vi "Search_comm_map_and_interrogate.vi"(7 "array of registers":T2[](array[typedef]) {"Cluster"."Mode" items=["None", "MODBUS", "HART", "Profibus DP", "Profibus PA", "Fieldbus", "DeviceNET"]}, 8 "error in (no error)":errorcluster, 9 "Register name":string="Flow Calibration Factor", 11 "Protocol in":refnum<class "Protocol.lvclass">) -> (0 "error out":errorcluster, 3 "Protocol out":refnum<class "Protocol.lvclass">, 4 "output cluster":T1)   [LabVIEW 2016]
uses:
  Typedef/comm_variable_definition.ctl
  Typedef/Comm_mode_and_address_type.ctl
  Typedef/Comm_mode_type_combo.ctl
  Protocol Class/Protocol.lvclass
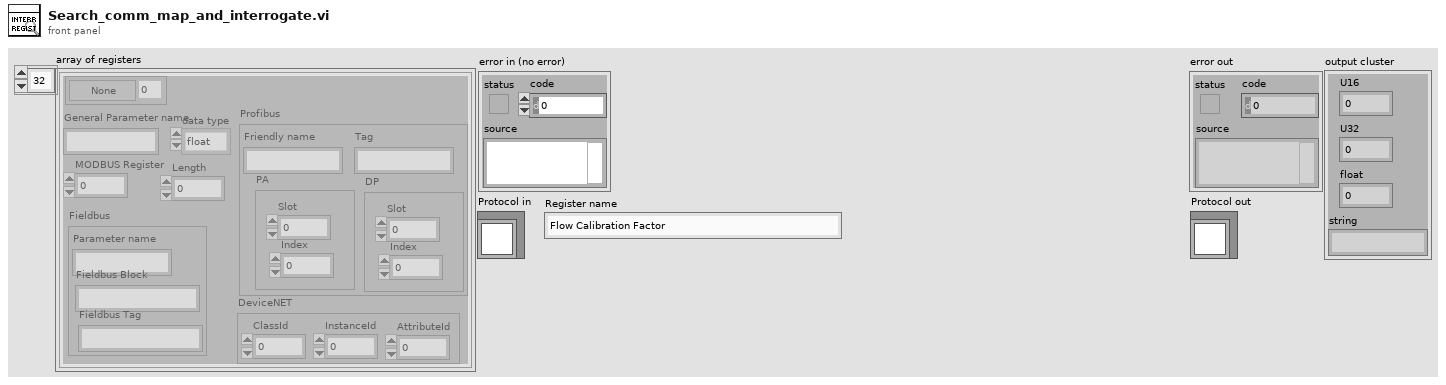
[diagram p1: front panel]
types:
  T1 = cluster{"U16":u16, "U32":u32, "float":sgl, "string":string}
  T2 = typedef "comm_variable_definition.ctl" = cluster{"General Parameter name":string, "MODBUS Register":i32, "Profibus":cluster{"Friendly name":string, "PA":cluster{"Slot":i32, "Index":i32}, "DP":cluster{"Slot":i32, "Index":i32}, "Tag":string}, "Fieldbus":cluster{"Parameter name":string, "Fieldbus Block":string, "Fieldbus Tag":string}, "data type":enum16{"float", "UINT", "UINT32", "STRING"}, "DeviceNET":cluster{"ClassId":u16, "InstanceId":u16, "AttributeId":u8}, "Cluster":T3, "Length":i32}
  T3 = typedef "Comm_mode_and_address_type.ctl" = cluster{"address":i32, "Mode":T4}
  T4 = typedef "Comm_mode_type_combo.ctl" = u16
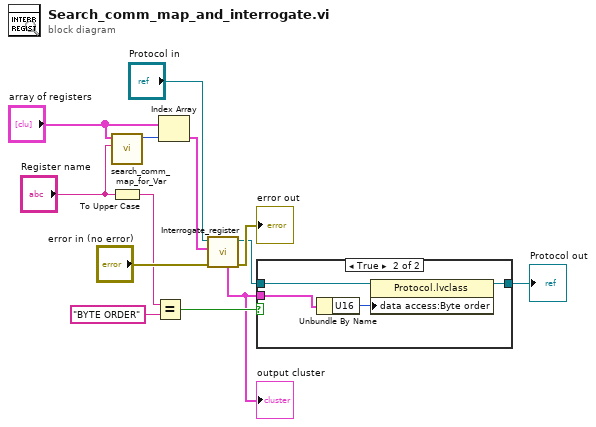
[diagram p0: block diagram]
diagram:
  n1 = call "search_comm_map_for_Var.vi"("Parameter"="Register name", "Comm variable definitions"="array of registers") -> ("index"=w13:i32)  [unwired: 8 in, 1 out]
  n2 = To Upper Case(1:"Register name") -> (0:w6:string)
  n3 = Equal?(x=w6, y="BYTE ORDER") -> (x = y?=w4:bool)
  n4 = Index Array(array="array of registers", index=w13) -> (element=w12:T2)
  n5 = call-dynamic "Interrogate_register.vi"("error in (no error)"="error in (no error)", "Register mutli-protocol location"=w12, "Protocol in"="Protocol in") -> ("error out"=→"error out":errorcluster, "Protocol out"=w3:refnum<class "Protocol.lvclass">, "output cluster"=w2:T1)  [unwired: 4 in, 2 out]
  "output cluster" <- w2
  n6 = case shown="True" w4 {
    tunnel: w3 -> [w14 w18]
    tunnel: w2 -> [_ w17]
    tunnel: [w14 w15] -> w1
    frame False {
    }
    frame True {
      n7 = Unbundle By Name(w17) -> ("U16"=w16:u16)
      n8 = property class="Protocol.lvclass"(reference=w18, "data access:Byte order"=w16) -> (reference out=w15:refnum<class "Protocol.lvclass">)  [unwired: 1 in, 1 out]
    }
  }
  "Protocol out" <- w1
